vi "WinCI Configure Project.vi"(8 "error in (no error)":errorcluster, 9 "configuration data in":string) -> (0 "error out":errorcluster, 1 "configuration data out":string, 2 "status message":string, 5 "dialog box cancelled?":bool)   [LabVIEW 2020, in "NI_SCC_WinCI.lvlib"]
uses:
  <vilib>/SourceControl/Providers/WinCI/NI_SCC_WinCI.lvlib
  <vilib>/SourceControl/Providers/WinCI/WinCI SCC Project Details.ctl
  <vilib>/SourceControl/support/SCCSup ConfigData Conv.ctl
  <vilib>/SourceControl/Providers/WinCI/WinCI Interface Functionality.ctl
  <vilib>/SourceControl/support/SCCSup Message Strings GLBL.vi
panel:
  out "result":i32
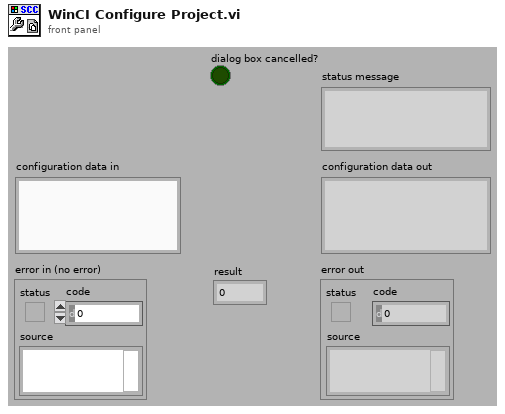
[diagram p1: front panel]
types:
  T1 = typedef "SCCSup ConfigData Conv.ctl" = enum16{"from config data", "to config data"}
  T2 = typedef "NI_SCC_WinCI.lvlib/WinCI SCC Project Details.ctl" = cluster{"user name":string, "project name":string, "local path":string, "database name":string}
  T3 = typedef "NI_SCC_WinCI.lvlib/WinCI Interface Functionality.ctl" = i32
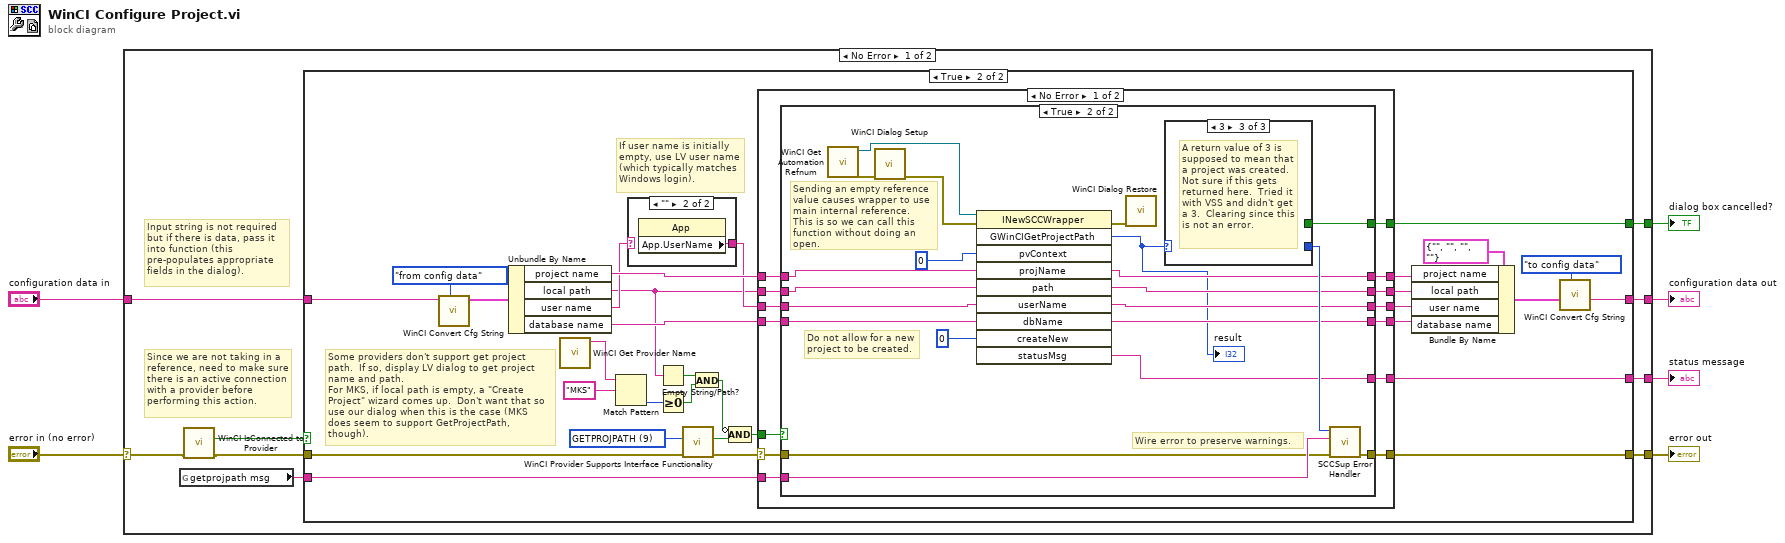
[diagram p0: block diagram]
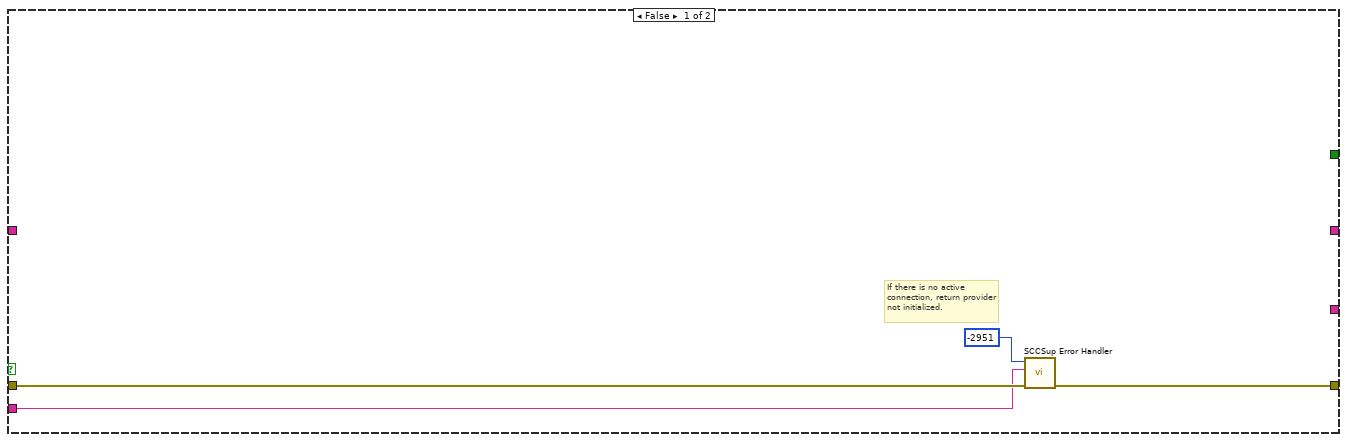
[diagram p2: hidden frame]
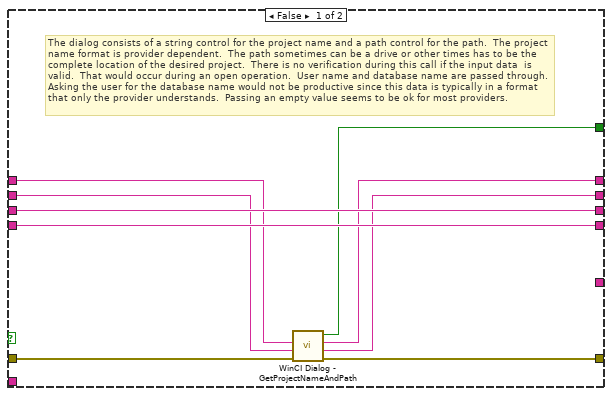
[diagram p4: hidden frame]
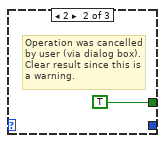
[diagram p6: hidden frame]
diagram:
  n1 = case shown="No Error" "error in (no error)" {
    selector: "error in (no error)" -> [w7 w100]
    tunnel: [w10 w100] -> w5
    tunnel: [w15 _] -> w4
    tunnel: [w14 _] -> w3
    tunnel: [w12 _] -> w2
    tunnel: "configuration data in" -> [w13 _]
    frame No Error {
      # "Input string is not required but if there is data, pass it into function (this pre-populates appropriate fields in the dialog)."
      # "Since we are not taking in a reference, need to make sure there is an active connection with a provider before performing this action."
      n2 = global read "SCCSup Message Strings GLBL.vi" "getprojpath msg"() -> (w11:string)
      n3 = call <vilib>:"WinCI IsConnected to Provider.vi"("error in (no error)"=w7) -> ("error out"=w8:errorcluster, "active connection?"=w9:bool)  [unwired: 9 out]
      n4 = case shown="True" w9 {
        tunnel: [_ w50] -> w15
        tunnel: [_ w49] -> w14
        tunnel: w13 -> [_ w26]
        tunnel: [_ w28] -> w12
        tunnel: w8 -> [w19 w21]
        tunnel: w11 -> [w18 w41]
        tunnel: [w16 w40] -> w10
        frame False {
          # "If there is no active connection, return provider not initialized."
          n5 = call <vilib>:"SCCSup Error Handler.vi"("error in (no error)"=w19, "operation message"=w18, "scc error code"=-2951 ("t")) -> ("error out"=w16:errorcluster)  [unwired: 1 in, 7 out]
        }
        frame True {
          w22 = T3 9 items=["REMOVE", "RENAME", "DIFF", "HISTORY", "PROPERTIES", "RUNSCC", "GETCOMMANDOPTIONS", "QUERYINFO", "GETEVENTS", "GETPROJPATH", "ADDFROMSCC", "COMMENTCHECKOUT", "COMMENTCHECKIN", "COMMENTADD", "COMMENTREMOVE", "TEXTOUT", "ADD_STORELATEST", "HISTORY_MULTIFILE", "IGNORECASE", "IGNORESPACE", "POPULATELIST", "COMMENTPROJECT", "DIFFALWAYS", "GET_NOUI", "REENTRANT"] ("interface functionality")
          # "If user name is initially empty, use LV user name (which typically matches Windows login)."
          # "Some providers don't support get project path.  If so, display LV dialog to get project name and path.\nFor MKS, if local path is empty, a \"Create Project\" wizard comes up.  Don't want that so use our dialog when this is the case (MKS does seem to support GetProjectPath, though)."
          n6 = call <vilib>:"WinCI Convert Cfg String.vi"("conversion action"=SCCSup_ConfigData_Conv."from config data", "config data in"=w26) -> ("project details out"=w27:T2)  [unwired: 1 in, 8 out]
          n7 = Unbundle By Name(w27) -> ("project name"=w43:string, "local path"=w31:string, "user name"=w39:string, "database name"=w42:string)
          n8 = call <vilib>:"WinCI Get Provider Name.vi"() -> ("provider name"=w20:string)  [unwired: 1 in, 10 out]
          n9 = Match Pattern(string=w20, regular expression="MKS") -> (offset past match=w36:i32)  [unwired: 4 out]
          n10 = case shown="\"\"" w39 {
            selector: w39 -> [w51 _]
            tunnel: [w51 w52] -> w38
            frame Default {
            }
            frame "" {
              n11 = property class="App"() -> ("App.UserName"=w52:string)  [unwired: 2 in, 2 out]
            }
          }
          n12 = Empty String/Path?(string/path=w31) -> (empty?=w34:bool)
          n13 = Greater Or Equal To 0?(x=w36) -> (x >= 0?=w33:bool)
          n14 = call <vilib>:"WinCI Provider Supports Interface Functionality.vi"("error in (no error)"=w21, "interface functionality"=w22) -> ("error out"=w23:errorcluster, "provider supports?"=w24:bool)  [unwired: 8 out]
          n15 = And(x=w34, y=w33) -> (x .and. y?=w32:bool)
          n16 = Compound Arithmetic op=AND(invert w32, w24) -> (w35:bool)
          n17 = case shown="No Error" w23 {
            selector: w23 -> [w54 w99]
            tunnel: [w66 _] -> w50
            tunnel: [w65 _] -> w49
            tunnel: [w64 _] -> w48
            tunnel: [w63 _] -> w47
            tunnel: [w62 _] -> w46
            tunnel: [w61 _] -> w44
            tunnel: w43 -> [w60 _]
            tunnel: w31 -> [w59 _]
            tunnel: w38 -> [w58 _]
            tunnel: w42 -> [w57 _]
            tunnel: w41 -> [w56 _]
            tunnel: [w55 w99] -> w40
            tunnel: w35 -> [w53 _]
            frame No Error {
              n18 = case shown="True" w53 {
                tunnel: [_ w85] -> w66
                tunnel: [w71 w96] -> w65
                tunnel: [w74 w83] -> w64
                tunnel: [w68 w81] -> w63
                tunnel: [w75 w84] -> w62
                tunnel: [w67 w82] -> w61
                tunnel: w60 -> [w70 w90]
                tunnel: w59 -> [w69 w89]
                tunnel: w58 -> [w74 w88]
                tunnel: w57 -> [w75 w87]
                tunnel: w56 -> [_ w95]
                tunnel: [w72 w93] -> w55
                tunnel: w54 -> [w73 w92]
                frame False {
                  # "The dialog consists of a string control for the project name and a path control for the path.  The project name format is provider dependent.  The path sometimes can be a drive or other times has to be the complete location of the desired project.  There is no verification during this call if the input data  is valid.  That would occur during an open operation.  User name and database name are passed through.  Asking the user for the database name would not be productive since this data is typically in a format that only the provider understands.  Passing an empty value seems to be ok for most providers."
                  n19 = call <vilib>:"WinCI Dialog - GetProjectNameAndPath.vi"("error in (no error)"=w73, "project path in"=w69, "project name in"=w70) -> ("error out"=w72:errorcluster, "project path out"=w67:string, "project name out"=w68:string, "cancelled?"=w71:bool)  [unwired: 5 out]
                }
                frame True {
                  # "Wire error to preserve warnings."
                  # "Sending an empty reference value causes wrapper to use main internal reference.  This is so we can call this function without doing an open."
                  # "Do not allow for a new project to be created."
                  n20 = call <vilib>:"WinCI Get Automation Refnum.vi"() -> ("error out"=w77:errorcluster, "automation refnum"=w80:refnum<k7>)  [unwired: 10 out]
                  n21 = call <vilib>:"WinCI Dialog Setup.vi"("error in"=w77) -> ("error out"=w78:errorcluster)  [unwired: 10 out]
                  n22 = invoke class="INewSCCWrapper" method="GWinCIGetProjectPath"(reference=w80, error in=w78, "pvContext"=u32 0, "projName"=w90, "path"=w89, "userName"=w88, "dbName"=w87, "createNew"=0) -> (error out=w76:errorcluster, "GWinCIGetProjectPath"=w79:i32, "projName"=w81:string, "path"=w82:string, "userName"=w83:string, "dbName"=w84:string, "statusMsg"=w85:string)  [unwired: 2 in, 3 out]
                  "result" <- w79
                  n23 = call <vilib>:"WinCI Dialog Restore.vi"("error in"=w76) -> ()  [unwired: 11 out]
                  n24 = case shown="3" w79 {
                    selector: w79 -> [w97 _ _]
                    tunnel: [w97 _ _] -> w94
                    tunnel: [_ TRUE _] -> w96
                    frame Default {
                    }
                    frame 2 {
                      # "Operation was cancelled by user (via dialog box).  Clear result since this is a warning."
                    }
                    frame 3 {
                      # "A return value of 3 is supposed to mean that a project was created.  Not sure if this gets returned here.  Tried it with VSS and didn't get a 3.  Clearing since this is not an error."
                    }
                  }
                  n25 = call <vilib>:"SCCSup Error Handler.vi"("error in (no error)"=w92, "operation message"=w95, "scc error code"=w94) -> ("error out"=w93:errorcluster)  [unwired: 1 in, 7 out]
                }
              }
            }
            frame Error {
            }
          }
          n26 = Bundle By Name(cluster=T2 {"user name"="", "project name"="", "local path"="", "database name"=""} ("returned project details"), "project name"=w47, "local path"=w44, "user name"=w48, "database name"=w46) -> (w29:T2)
          n27 = call <vilib>:"WinCI Convert Cfg String.vi"("conversion action"=SCCSup_ConfigData_Conv."to config data", "project details in"=w29) -> ("config data out"=w28:string)  [unwired: 1 in, 8 out]
        }
      }
    }
    frame Error {
    }
  }
  "error out" <- w5
  "status message" <- w4
  "dialog box cancelled?" <- w3
  "configuration data out" <- w2
